vi "MTMount_getEvent_mountWarning.vi"(8 "error in (no error)":errorcluster, 11 "logevent_mountWarning_Ctl":T1) -> (0 "error out":errorcluster, 2 "function return":i32, 3 "logevent_mountWarning_Ctl out":T1)   [LabVIEW 2018, in "SALLV_MTMount.lvlib"]
doc: "int MTMount_shm_getEvent_mountWarningLV(MTMount_logevent_mountWarningLV *logevent_mountWarning_Ctl );"
uses:
  SALLV_MTMount.lvlib
  DataTypes/logevent_mountWarning.ctl
  SALLV_MTMount.so
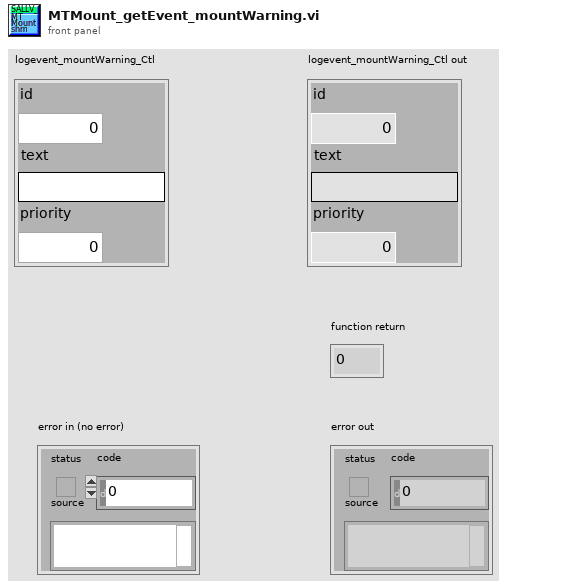
[diagram p1: front panel]
types:
  T1 = typedef "SALLV_MTMount.lvlib/logevent_mountWarning.ctl" = cluster{"id":i32, "text":string, "priority":i32}
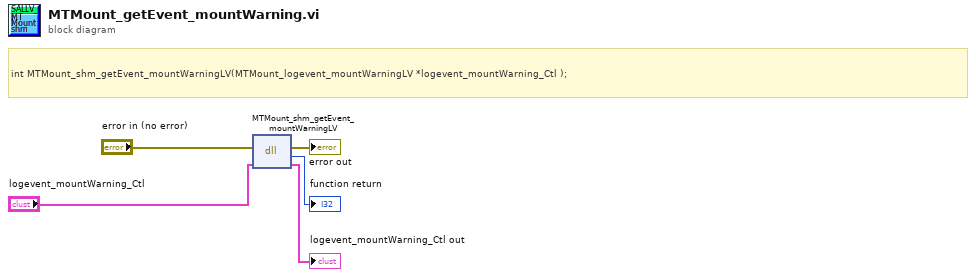
[diagram p0: block diagram]
diagram:
  # "int MTMount_shm_getEvent_mountWarningLV(MTMount_logevent_mountWarningLV *logevent_mountWarning_Ctl );"
  n1 = dll-call lib="home/ttsai/Document/salApiMTMount/SALLV_MTMount/SALLV_MTMount.*" fn="MTMount_shm_getEvent_mountWarningLV"(error in="error in (no error)", "logevent_mountWarning_Ctl"="logevent_mountWarning_Ctl") -> (error out=→"error out":errorcluster, →"function return":i32, "logevent_mountWarning_Ctl"=→"logevent_mountWarning_Ctl out":T1)  [unwired: 2 in, 1 out]
